vi "Helmholtz2D_Cal Coef Mtrx.vi"(8 "Boundary Condition":cluster{"type":T2, "Value":dbl[]}[](array[cluster]) {"type" items=["Dirichlet", "Neumann"]}, 9 "Domain":T3={"x"={"start x"=0.0, "end x"=1.0, "# of x-points"=11}, "y"={"start y"=0.0, "end y"=1.0, "# of y-points"=11}}, 10 "a":dbl, 11 "k":dbl=1.0) -> (0 "D":T1, 1 "C":T1, 2 "D'":T1, 3 "C'":T1)   [LabVIEW 2017, in "NI_PDE.lvlib"]
uses:
  <vilib>/gmath/NI_PDE.lvlib
  <vilib>/Analysis/Matrix/Datatypes/RealMatrix.ctl
  <vilib>/gmath/pde.llb/Common/PDE_BC Type.ctl
  <vilib>/Analysis/7linalg.llb/Create Special Real Matrix.vi
  <vilib>/Analysis/Matrix/Numeric/Multiply/Multiply - RM,R.vi
  <vilib>/Analysis/Matrix/Numeric/Multiply/Multiply - R,RM.vi
  <vilib>/Analysis/Matrix/Numeric/Add/Add - RM,RM.vi
  <vilib>/Analysis/Matrix/NI_Matrix.lvlib
  <vilib>/Analysis/NI_AALPro.lvlib
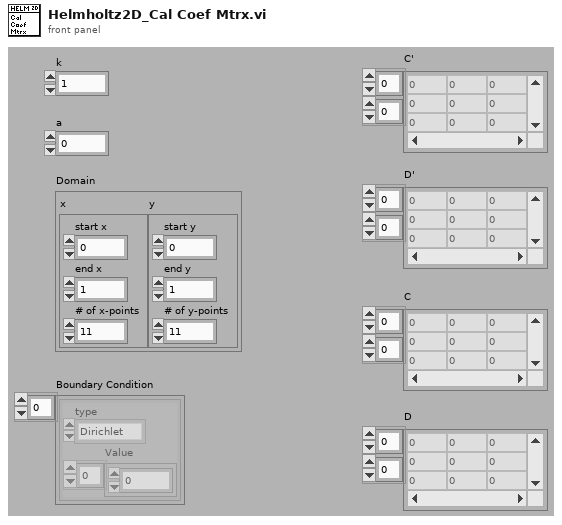
[diagram p1: front panel]
types:
  T1 = typedef "NI_Matrix.lvlib/RealMatrix.ctl" = dbl[][]
  T2 = typedef "NI_PDE.lvlib/PDE_BC Type.ctl" = i32
  T3 = cluster{"x":cluster{"start x":dbl, "end x":dbl, "# of x-points":i32}, "y":cluster{"start y":dbl, "end y":dbl, "# of y-points":i32}}
  T4 = enum32{"Identity", "Diagonal", "Toepliz", "Vandermonde", "Companion"}
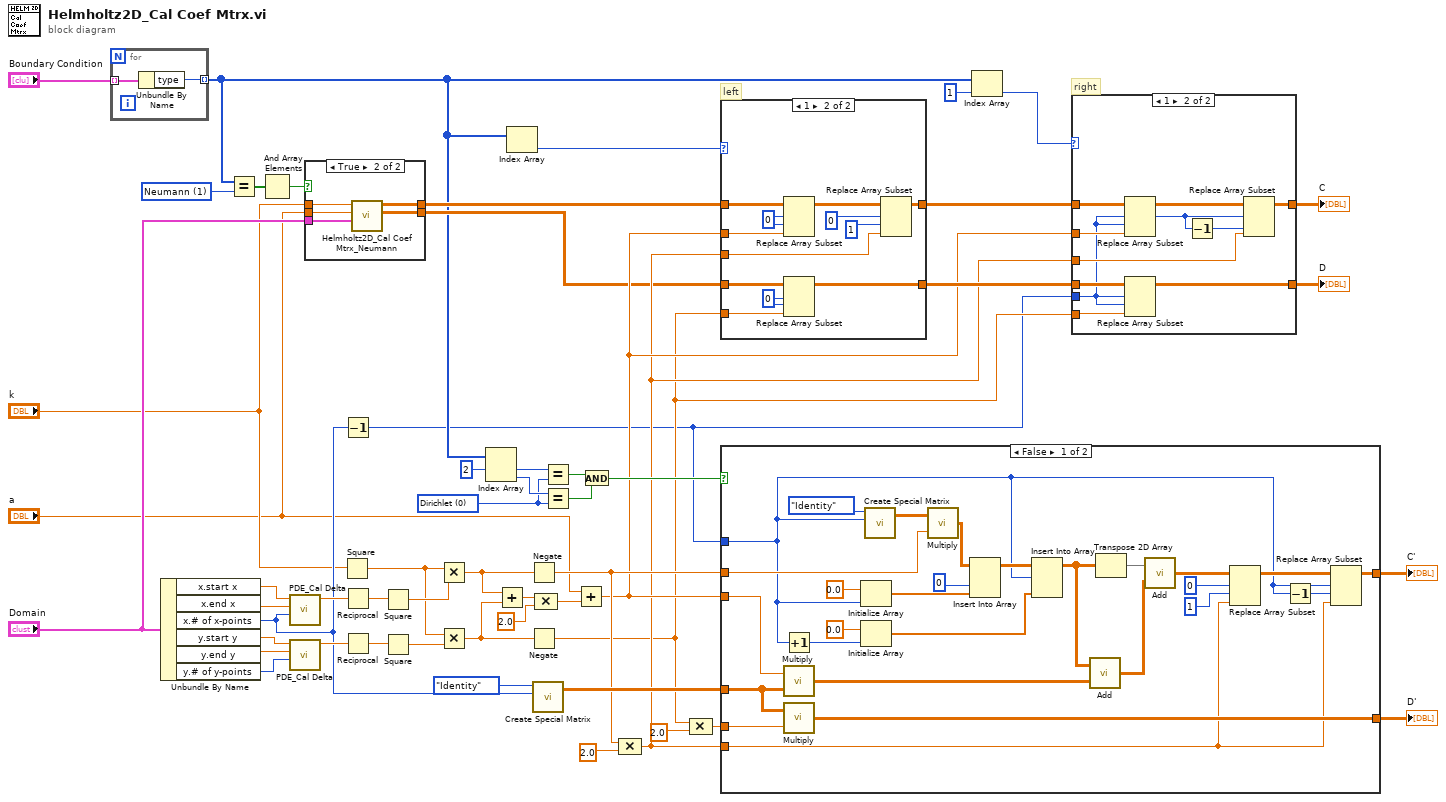
[diagram p0: block diagram]
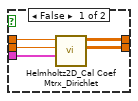
[diagram p2: hidden frame]
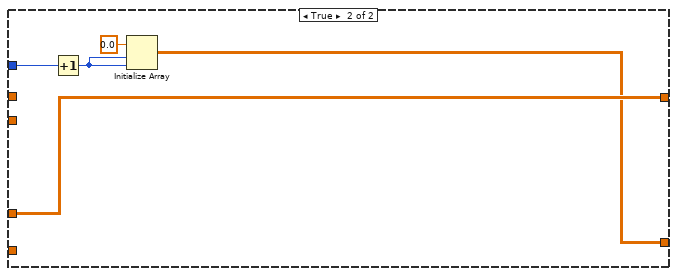
[diagram p3: hidden frame]
diagram:
  w5 = T2 0 items=["Dirichlet", "Neumann"] ("x")
  w22 = T2 1 items=["Dirichlet", "Neumann"] ("type")
  # "right"
  # "left"
  n1 = for {
    tunnel: "Boundary Condition" -> [w56] mode=indexing
    tunnel: [w55] -> w18 mode=indexing
    n2 = Unbundle By Name(w56) -> ("type"=w55:T2)
  }
  n3 = Unbundle By Name("Domain") -> ("x.start x"=w17:dbl, "x.end x"=w16:dbl, "x.# of x-points"=w10:i32, "y.start y"=w14:dbl, "y.end y"=w15:dbl, "y.# of y-points"=w13:i32)
  n4 = Equal?(x=w18, y=w22) -> (x = y?=w21:bool[])
  n5 = And Array Elements(Boolean array=w21) -> (logical AND=w19:bool)
  n6 = call <vilib>:"PDE_Cal Delta.vi"("# of points"=w10, "end"=w16, "start"=w17) -> ("delta"=w12:dbl)  [unwired: 8 out]
  n7 = call <vilib>:"PDE_Cal Delta.vi"("# of points"=w13, "end"=w15, "start"=w14) -> ("delta"=w11:dbl)  [unwired: 8 out]
  n8 = case shown="True" w19 {
    tunnel: "a" -> [w58 w63]
    tunnel: "k" -> [w59 w64]
    tunnel: [w60 w66] -> w28
    tunnel: [w61 w65] -> w27
    tunnel: "Domain" -> [w57 w62]
    frame False {
      n9 = call <vilib>:"Helmholtz2D_Cal Coef Mtrx_Dirichlet.vi"("Domain"=w57, "a"=w58, "k"=w59) -> ("D"=w61:T1, "C"=w60:T1)  [unwired: 7 out]
    }
    frame True {
      n10 = call <vilib>:"Helmholtz2D_Cal Coef Mtrx_Neumann.vi"("Domain"=w62, "a"=w63, "k"=w64) -> ("D"=w65:T1, "C"=w66:T1)  [unwired: 7 out]
    }
  }
  n11 = Square(x="k") -> (x^2=w50:dbl)
  n12 = Decrement(x=w10) -> (x-1=w9:i32)
  n13 = Reciprocal(x=w12) -> (1/x=w2:dbl)
  n14 = Reciprocal(x=w11) -> (1/x=w1:dbl)
  n15 = Square(x=w2) -> (x^2=w51:dbl)
  n16 = Square(x=w1) -> (x^2=w52:dbl)
  n17 = Multiply(x=w50, y=w51) -> (x*y=w36:dbl)
  n18 = Multiply(x=w50, y=w52) -> (x*y=w48:dbl)
  n19 = Index Array(array=w18, index #1=2 ("index")) -> (element #1=w40:T2, element #2=w6:T2)  [unwired: 1 in]
  n20 = Add(x=w36, y=w48) -> (x+y=w54:dbl)
  n21 = Index Array(array=w18) -> (element=w47:T2)  [unwired: 1 in]
  n22 = Negate(x=w36) -> (-x=w35:dbl)
  n23 = Negate(x=w48) -> (-x=w30:dbl)
  n24 = call-poly <vilib>:"Create Special Matrix.vi"("matrix type"=T4."Identity", "matrix size"=w10) -> ("Special Matrix"=w41:T1)  [unwired: 2 in, 2 out]
  n25 = Compound Arithmetic op=MULTIPLY(w54, 2.0 ("y")) -> (w53:dbl)
  n26 = Equal?(x=w40, y=w5) -> (x = y?=w39:bool)
  n27 = Equal?(x=w6, y=w5) -> (x = y?=w38:bool)
  n28 = Add(x="a", y=w53) -> (x+y=w33:dbl)
  n29 = And(x=w39, y=w38) -> (x .and. y?=w37:bool)
  n30 = Compound Arithmetic op=MULTIPLY(w35, 2.0 ("y")) -> (w32:dbl)
  n31 = Compound Arithmetic op=MULTIPLY(w30, 2.0 ("y")) -> (w29:dbl)
  n32 = case shown="1" w47 {
    tunnel: w28 -> [w68 w80]
    tunnel: [w68 w76] -> w46
    tunnel: w33 -> [_ w77]
    tunnel: [w67 w71] -> w34
    tunnel: w32 -> [_ w73]
    tunnel: w30 -> [_ w70]
    tunnel: w27 -> [w67 w69]
    frame 0, Default {
    }
    frame 1 {
      w72 = 0 ("index (row)")
      w79 = 0 ("index (row)")
      n33 = Replace Array Subset(array=w80, new element=w77, index (row)=w79, index (col)=w79) -> (w78:T1)
      n34 = Replace Array Subset(array=w69, new element=w70, index (row)=w72, index (col)=w72) -> (w71:T1)
      n35 = Replace Array Subset(array=w78, new element=w73, index (row)=0, index (col)=1 ("index (row)")) -> (w76:T1)
    }
  }
  n36 = case shown="False" w37 {
    tunnel: w33 -> [w94 _]
    tunnel: [w83 w109] -> w25
    tunnel: w29 -> [w93 _]
    tunnel: w35 -> [w91 _]
    tunnel: w9 -> [w81 w108]
    tunnel: w32 -> [w82 _]
    tunnel: [w85 w112] -> w26
    tunnel: w41 -> [w84 w112]
    frame False {
      n37 = Increment(x=w81) -> (x+1=w95:i32)
      n38 = call-poly <vilib>:"Multiply.vi"("Real Matrix A"=w84, "Real Scalar c"=w94) -> ("c * A"=w92:T1)
      n39 = call-poly <vilib>:"Multiply.vi"("Real Scalar c"=w93, "Real Matrix A"=w84) -> ("A * c"=w83:T1)
      n40 = Initialize Array(0.0 ("element"), w81) -> (w103:dbl[])
      n41 = Initialize Array(0.0 ("element"), w95) -> (w99:dbl[])
      n42 = call-poly <vilib>:"Create Special Matrix.vi"("matrix type"=T4."Identity", "matrix size"=w81) -> ("Special Matrix"=w106:T1)  [unwired: 2 in, 2 out]
      n43 = call-poly <vilib>:"Multiply.vi"("Real Scalar c"=w91, "Real Matrix A"=w106) -> ("A * c"=w104:T1)
      n44 = Insert Into Array(array=w104, index (col)=0 ("disabled index (col)"), new element=w103) -> (w101:T1)  [unwired: 1 in]
      n45 = Insert Into Array(array=w101, index (row)=w81, new element=w99) -> (w98:T1)  [unwired: 1 in]
      n46 = call-poly <vilib>:"Add.vi"("Real Matrix B"=w92, "Real Matrix A"=w98) -> ("A + B"=w97:T1)
      n47 = Transpose 2D Array(2D array=w98) -> (transposed array=w96:T1)
      n48 = call-poly <vilib>:"Add.vi"("Real Matrix B"=w97, "Real Matrix A"=w96) -> ("A + B"=w86:T1)
      n49 = Replace Array Subset(array=w86, new element=w82, index (row)=0 ("disabled index (col)"), index (col)=1 ("disabled index (col)")) -> (w88:T1)
      n50 = Decrement(x=w81) -> (x-1=w87:i32)
      n51 = Replace Array Subset(array=w88, new element=w82, index (row)=w81, index (col)=w87) -> (w85:T1)
    }
    frame True {
      n52 = Increment(x=w108) -> (x+1=w111:i32)
      n53 = Initialize Array(0.0 ("element"), w111, w111) -> (w109:dbl[][])
    }
  }
  "C'" <- w26
  "D'" <- w25
  n54 = Index Array(array=w18, index=1) -> (element=w45:T2)
  n55 = case shown="1" w45 {
    tunnel: w46 -> [w114 w124]
    tunnel: [w114 w121] -> w24
    tunnel: w33 -> [_ w122]
    tunnel: w9 -> [_ w116]
    tunnel: w34 -> [w113 w118]
    tunnel: [w113 w117] -> w23
    tunnel: w32 -> [_ w119]
    tunnel: w30 -> [_ w115]
    frame 0, Default {
    }
    frame 1 {
      n56 = Replace Array Subset(array=w124, new element=w122, index (row)=w116, index (col)=w116) -> (w123:T1)
      n57 = Replace Array Subset(array=w118, new element=w115, index (row)=w116, index (col)=w116) -> (w117:T1)
      n58 = Decrement(x=w116) -> (x-1=w120:i32)
      n59 = Replace Array Subset(array=w123, new element=w119, index (row)=w116, index (col)=w120) -> (w121:T1)
    }
  }
  "D" <- w23
  "C" <- w24
